vi "Read Multiple Digital Ports.vi"() -> ()   [LabVIEW 2020]
uses:
  <instrlib>/BDAQ-6104/Public/Data/Read Multiple Digital Channels.vi
  <instrlib>/BDAQ-6104/BDAQ-6104.lvlib
panel:
  out "Digital Pins":bool[](array[boolean])
  in  "Digital Pin":T1(array[ring])=[enum."Digital Pin 0", enum."Digital Pin 1", enum."Digital Pin 2", enum."Digital Pin 3"]
  in  "VISA resource name":refnum<visa-resource-name>
  # "Reads the current state of the pins specified \nin the digital pin array."
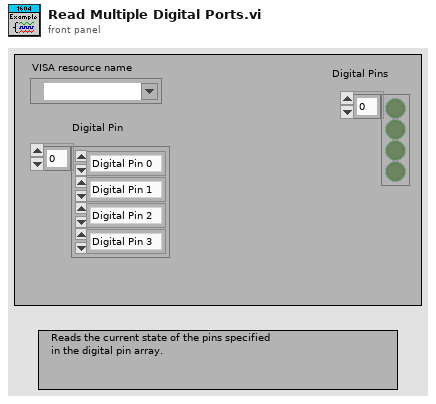
[diagram p1: front panel]
types:
  T1 = enum16{"Digital Pin 0", "Digital Pin 1", "Digital Pin 2", "Digital Pin 3"}[]
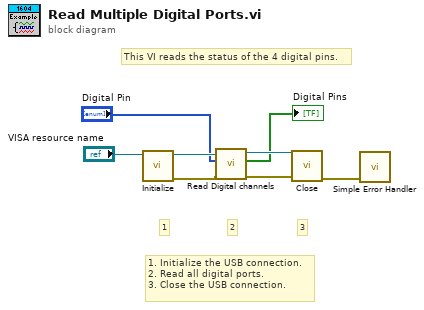
[diagram p0: block diagram]
diagram:
  # "This VI reads the status of the 4 digital pins."
  # "1. Initialize the USB connection.\n2. Read all digital ports.\n3. Close the USB connection."
  # "3"
  # "2"
  # "1"
  n1 = call <instrlib>:"Initialize.vi"("VISA resource name"="VISA resource name") -> ("error out"=w7:errorcluster, "VISA resource name out"=w6:refnum<visa-resource-name>)  [unwired: 9 in]
  n2 = call-poly <instrlib>:"Read Digital channels.vi"("error in (no error)"=w7, "Digital Pin"="Digital Pin", "VISA resource name"=w6) -> ("error out"=w5:errorcluster, "Array"=→"Digital Pins":bool[], "VISA resource name out"=w4:refnum<visa-resource-name>)  [unwired: 6 in]
  n3 = call <instrlib>:"Close.vi"("error in (no error)"=w5, "VISA resource name"=w4) -> ("error out"=w1:errorcluster)  [unwired: 9 in]
  n4 = call <vilib>:"Simple Error Handler.vi"("error in (no error)"=w1) -> ()  [unwired: 4 in, 5 out]
